vi "csv.vi"(7 "LabVIEW Web Service Request":refnum<class "Web Request.lvclass">, 10 "end":dbl, 11 "start":dbl) -> (3 "Data":string)   [LabVIEW 2017]
uses:
  <vilib>/wsapi/Web Request.lvclass
  private/GlobalVariable.vi
panel:
  out "error out":errorcluster
  out "#Output":i32
  out "#Input":i32
  # "Use the Web Service Request input terminal to call the VIs on the Web Services palette. Do not remove it from the connector pane unless you don't need access to the palette."
  # "Each additional control wired to the connector pane will be available as an input in the URL. To include an indicator in terminal-mode output (the default setting), it must also be wired to the connector pane."
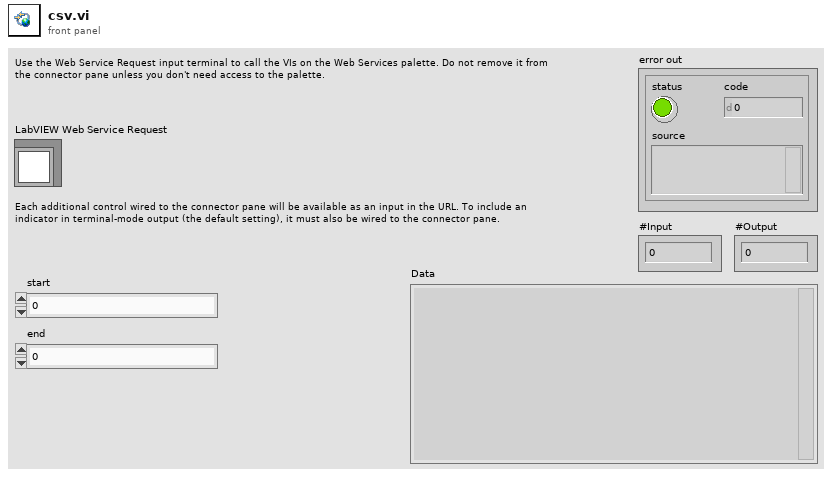
[diagram p1: front panel]
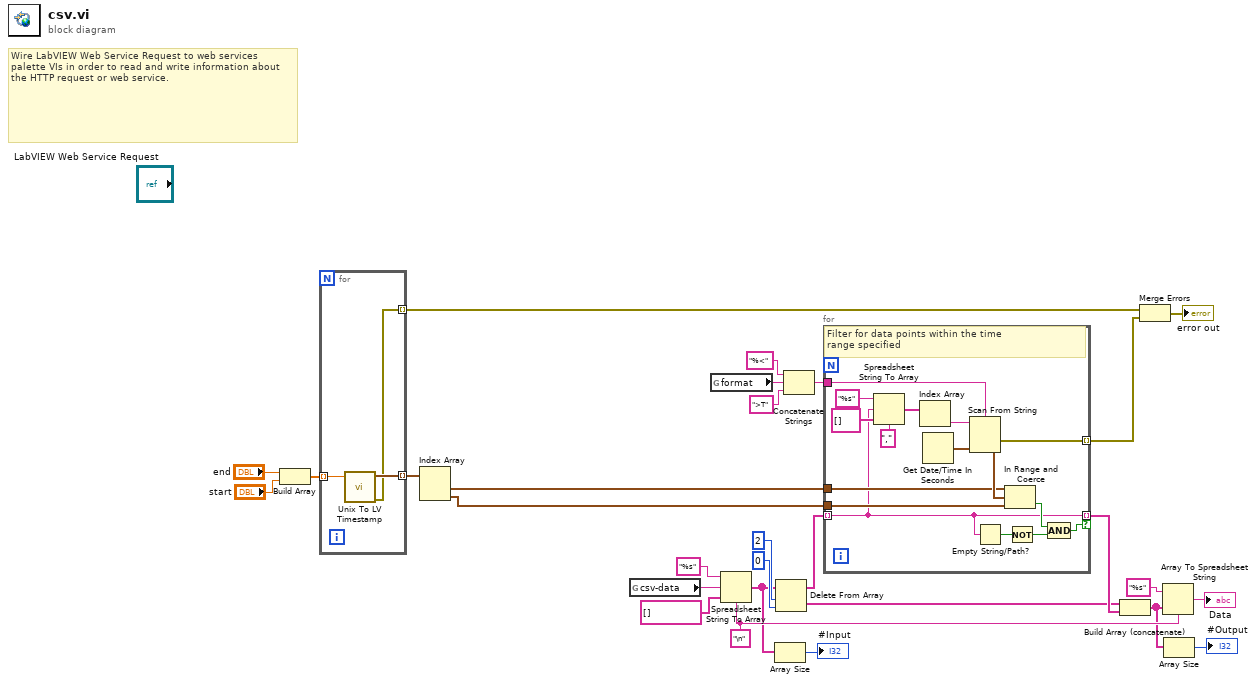
[diagram p0: block diagram]
diagram:
  w17 = "\n" ("format string")
  # "Wire LabVIEW Web Service Request to web services palette VIs in order to read and write information about the HTTP request or web service."
  n1 = Build Array("end", "start") -> (w13:dbl[])
  n2 = for {
    tunnel: w13 -> [w31] mode=indexing
    tunnel: [w30] -> w12 mode=indexing
    tunnel: [w29] -> w9 mode=indexing
    n3 = call "Unix To LV Timestamp.vi"("UTC Unix Offset"=w31) -> ("error out"=w29:errorcluster, "TimeStamp"=w30:timestamp)  [unwired: 9 in]
  }
  n4 = Index Array(array=w12) -> (element #1=w10:timestamp, element #2=w11:timestamp)  [unwired: 2 in]
  n5 = global read "GlobalVariable.vi" "csv-data"() -> (w28:string)
  n6 = global read "GlobalVariable.vi" "format"() -> (w18:string)
  n7 = Spreadsheet String To Array(delimiter (Tab)=w17, format string="%s", spreadsheet string=w28, array type (2D Dbl)=string[] []) -> (array=w5:string[])
  n8 = Array Size(array=w5) -> (size(s)=→"#Input":i32)
  n9 = Delete From Array(array=w5, length=2 ("index"), index=0) -> (deleted portion=w7:string[], array with subset deleted=w6:string[])
  n10 = Concatenate Strings("%<" ("format string"), w18, ">T" ("input 2")) -> (w19:string)
  n11 = for {
    tunnel: w6 -> [w34] mode=indexing
    tunnel: [w34] -> w25 mode=indexing if=w36
    tunnel: [w42] -> w22 mode=indexing
    tunnel: w19 -> [w41]
    tunnel: w11 -> [w38]
    tunnel: w10 -> [w35]
    # "Filter for data points within the time \nrange specified"
    n12 = Spreadsheet String To Array(delimiter (Tab)="," ("format string"), format string="%s", spreadsheet string=w34, array type (2D Dbl)=string[] []) -> (array=w44:string[])
    n13 = Index Array(array=w44) -> (element=w43:string)  [unwired: 1 in]
    n14 = Get Date/Time In Seconds() -> (seconds since 1Jan1904=w40:timestamp)
    n15 = Scan From String(format string=w41, input string=w43, default 1=w40) -> (error out=w42:errorcluster, output 1=w39:timestamp)  [unwired: 2 in, 2 out]
    n16 = Empty String/Path?(string/path=w34) -> (empty?=w33:bool)
    n17 = In Range and Coerce(upper limit=w35, x=w39, lower limit=w38) -> (In Range?=w37:bool)  [unwired: 1 out]
    n18 = Not(x=w33) -> (.not. x?=w32:bool)
    n19 = Compound Arithmetic op=AND(w37, w32) -> (w36:bool)
  }
  n20 = Build Array (concatenate)(w7, w25) -> (w4:string[])
  n21 = Merge Errors(w9, w22) -> (→"error out":errorcluster)
  n22 = Array To Spreadsheet String(delimiter (Tab)=w17, array=w4, 3:"%s" ("format string")) -> (spreadsheet string=→"Data":string)
  n23 = Array Size(array=w4) -> (size(s)=→"#Output":i32)
